vi "half_min_ts.vi"() -> (0 "time stamp":timestamp)   [LabVIEW 2021]
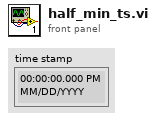
[diagram p1: front panel]
types:
  T1 = typedef "LVDateTimeRec.ctl" = cluster{"fractional second":dbl, "second":i32, "minute":i32, "hour":i32, "day of month":i32, "month":i32, "year":i32, "day of week":i32, "day of year":i32, "DST":i32}
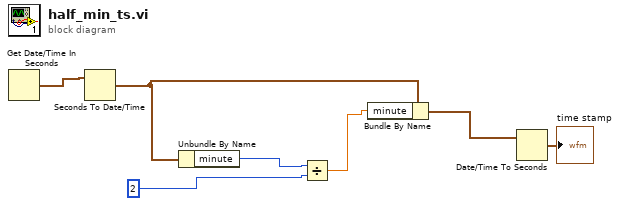
[diagram p0: block diagram]
diagram:
  n1 = Get Date/Time In Seconds() -> (seconds since 1Jan1904=w7:timestamp)
  n2 = Seconds To Date/Time(time stamp (now)=w7) -> (date time rec=w3:T1)  [unwired: 1 in]
  n3 = Unbundle By Name(w3) -> ("minute"=w6:i32)
  n4 = Divide(x=w6, y=2) -> (x/y=w4:dbl)
  n5 = Bundle By Name(cluster=w3, "minute"=w4) -> (w2:T1)
  n6 = Date/Time To Seconds(2:w2) -> (0:→"time stamp":timestamp)  [unwired: 1 in]
